vi "check control hz array.vi"(10 "count":u16, 11 "control hz array":dbl[][](array[numeric])) -> (3 "logical AND":bool)   [LabVIEW 2014]
panel:
  out "boolean":bool[](array[boolean])
  out "size":i32
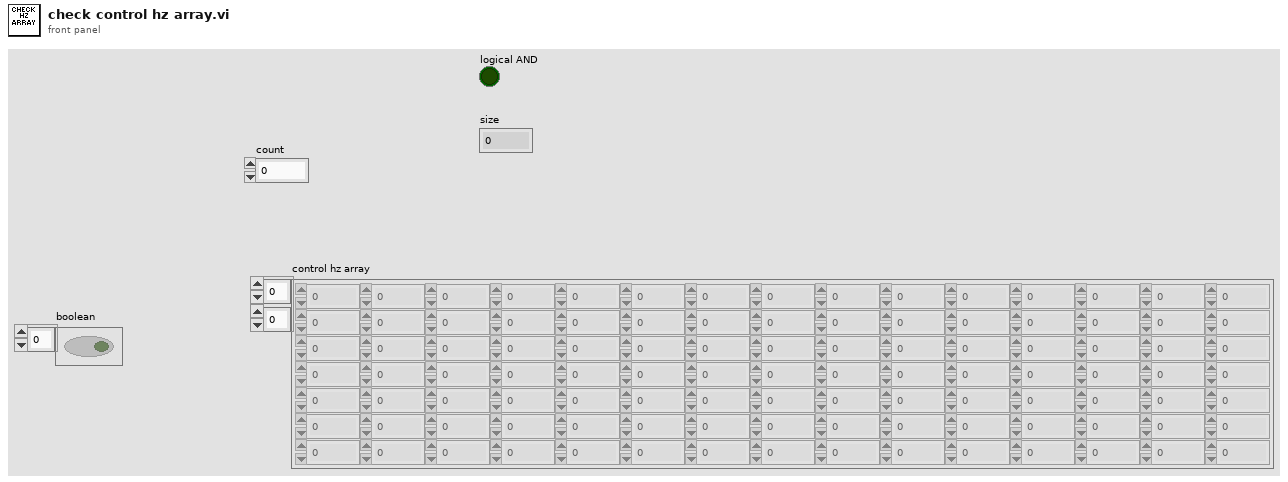
[diagram p1: front panel]
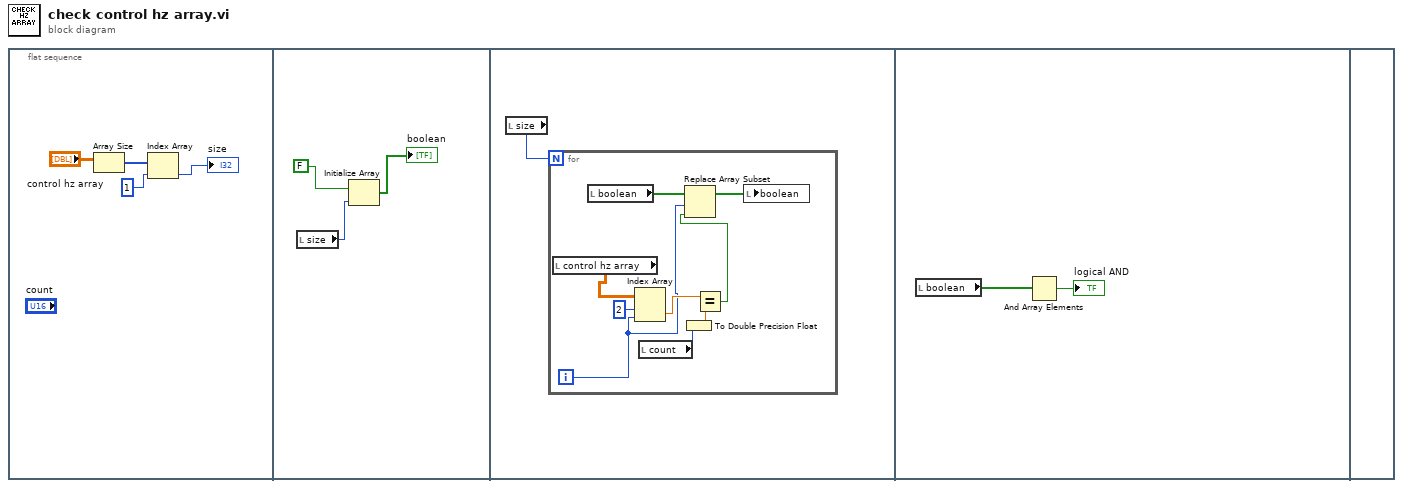
[diagram p0: block diagram]
diagram:
  n1 = flat-sequence {
    frame #0 {
      n2 = Array Size(array="control hz array") -> (size(s)=w3:i32[])
      n3 = Index Array(array=w3, index=1) -> (element=→"size":i32)
    }
    frame #1 {
      n4 = local read "size"() -> (w6:i32)
      n5 = Initialize Array(FALSE, w6) -> (→"boolean":bool[])
    }
    frame #2 {
      n6 = local read "size"() -> (w8:i32)
      n7 = for {
        N: w8 -> [_]
        i -> [w10]
        n8 = local read "control hz array"() -> (w16:dbl[][])
        n9 = local read "boolean"() -> (w17:bool[])
        n10 = Index Array(array=w16, index (row)=2, index (col)=w10) -> (element=w13:dbl)
        n11 = local read "count"() -> (w14:u16)
        n12 = To Double Precision Float(number=w14) -> (double precision float=w12:dbl)
        n13 = Equal?(x=w13, y=w12) -> (x = y?=w11:bool)
        n14 = Replace Array Subset(array=w17, new element=w11, index=w10) -> (w9:bool[])
        n15 = local write "boolean"(w9) -> ()
      }
    }
    frame #3 {
      n16 = local read "boolean"() -> (w19:bool[])
      n17 = And Array Elements(Boolean array=w19) -> (logical AND=→"logical AND":bool)
    }
    frame #4 {
    }
  }
